vi "Close TreeSelectionHierarchal.vi"(8 "error in (no error)":errorcluster, 11 "TreeHier in":refnum<class "TreeSelectionHierarchal.lvclass">) -> (0 "error out":errorcluster)   [LabVIEW 2015, in "TreeSelectionHierarchal.lvclass"]
uses:
  TreeSelectionHierarchal.lvclass
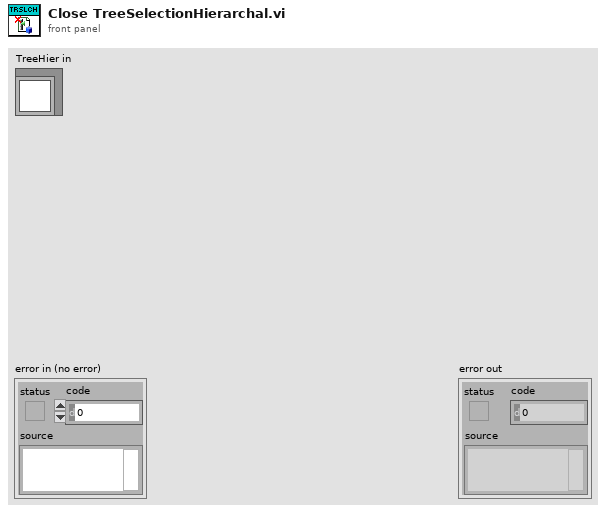
[diagram p1: front panel]
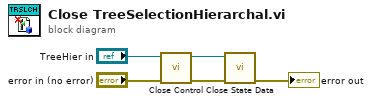
[diagram p0: block diagram]
diagram:
  n1 = call-dynamic "Close Control.vi"("error in (no error)"="error in (no error)", "Control in"="TreeHier in") -> ("error out"=w4:errorcluster, "Control out"=w1:refnum<class "TreeSelectionHierarchal.lvclass">)  [unwired: 8 in]
  n2 = call-dynamic "Close State Data.vi"("error in (no error)"=w4, "Control in"=w1) -> ("error out"=→"error out":errorcluster)  [unwired: 8 in, 1 out]
